vi "Ball Screw Control.vi"(6 "Target":bool, 7 "Axis":dbl, 8 "BotLimit":bool, 9 "TopLimit":bool, 10 "Closed Loop On/Off":bool, 11 "Ball Screw DevRef In":T1={"DeviceStatus"={"status"=FALSE, "code"=0, "source"=""}, "Type"=enum."PWM", "PWM"={"Digital Module"=enum."Digital Module 1", "PWM Channel"=enum."Invalid", "DeadBand"={"Name"="", "maxPositivePwm"=0, "minPositivePwm"=0, "centerPwm"=0, "maxNegativePwm"=0, "minNegativePwm"=0, "angularRange"=0}}, "CAN"={"Device Number"=0, "Control Mode"=enum."Percent VBus", "Semaphore"=refnum, "Max Vout"=12.0}, "Invert"=FALSE, "TransformRef"=refnum, "InvTransformRef"=refnum}) -> (2 "Motor Output":dbl, 3 "Ball Screw DevRef Out":T1={"DeviceStatus"={"status"=FALSE, "code"=0, "source"=""}, "Type"=enum."PWM", "PWM"={"Digital Module"=enum."Digital Module 1", "PWM Channel"=enum."Invalid", "DeadBand"={"Name"="", "maxPositivePwm"=0, "minPositivePwm"=0, "centerPwm"=0, "maxNegativePwm"=0, "minNegativePwm"=0, "angularRange"=0}}, "CAN"={"Device Number"=0, "Control Mode"=enum."Percent VBus", "Semaphore"=refnum, "Max Vout"=12.0}, "Invert"=FALSE, "TransformRef"=refnum, "InvTransformRef"=refnum})   [LabVIEW 2012]
uses:
  <vilib>/Rock Robotics/WPI/MotorControl/WPI_MotorControlDeviceRef.ctl
  <vilib>/Rock Robotics/SystemInterfaces/Typedef/FPGA_TypedefDigitalModule.ctl
  <vilib>/Rock Robotics/SystemInterfaces/DIO/FPGA_DIOPWMChannel.ctl
  <vilib>/Rock Robotics/WPI/PWM/WPI_PWMDeadband.ctl
  <vilib>/Rock Robotics/WPI/CAN/Jaguar/SubVIs/WPI_CANJaguar_ControlMode.ctl
  <vilib>/Rock Robotics/WPI/PWM/WPI_PWMTransform_ConPane.ctl
  <vilib>/Rock Robotics/WPI/CAN/Jaguar/SubVIs/WPI_CANJaguar_PositionReference.ctl
  Robot Global Data.vi
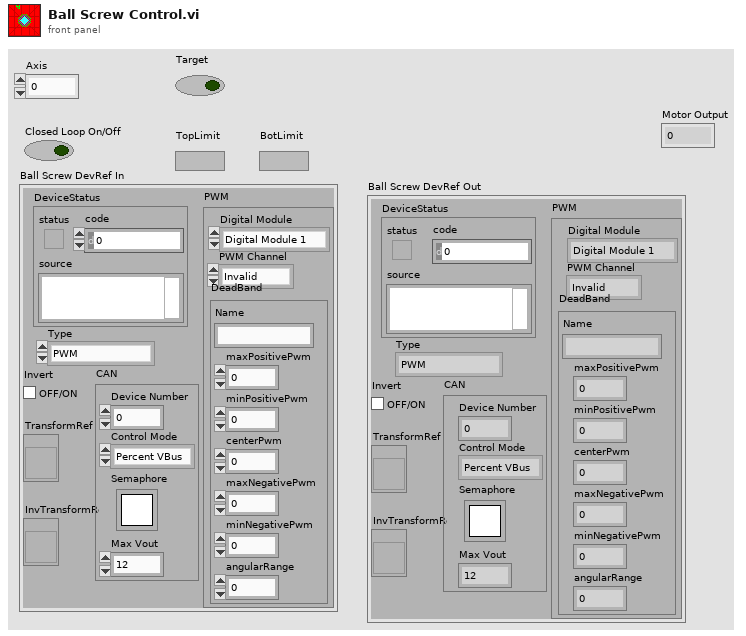
[diagram p1: front panel]
types:
  T1 = typedef "WPI_MotorControlDeviceRef.ctl" = cluster{"DeviceStatus":errorcluster, "Type":enum16{"PWM", "CAN"}, "PWM":cluster{"Digital Module":T2, "PWM Channel":T3, "DeadBand":T4}, "CAN":cluster{"Device Number":u8, "Control Mode":T5, "Semaphore":T6, "Max Vout":dbl}, "Invert":bool, "TransformRef":T7, "InvTransformRef":T7}
  T2 = typedef "FPGA_TypedefDigitalModule.ctl" = enum16{"Digital Module 1", "Digital Module 2"}
  T3 = typedef "FPGA_DIOPWMChannel.ctl" = enum8{"PWM 1", "PWM 2", "PWM 3", "PWM 4", "PWM 5", "PWM 6", "PWM 7", "PWM 8", "PWM 9", "PWM 10", "Invalid"}
  T4 = typedef "WPI_PWMDeadband.ctl" = cluster{"Name":string, "maxPositivePwm":i32, "minPositivePwm":i32, "centerPwm":i32, "maxNegativePwm":i32, "minNegativePwm":i32, "angularRange":u16}
  T5 = typedef "WPI_CANJaguar_ControlMode.ctl" = enum8{"Percent VBus", "Current", "Speed", "Position", "Voltage"}
  T6 = typedef "Semaphore RefNum" = refnum<k1>
  T7 = typedef "WPI_PWMTransform_ConPane.ctl" = refnum<vi>
  T8 = typedef "WPI_CANJaguar_PositionReference.ctl" = u8
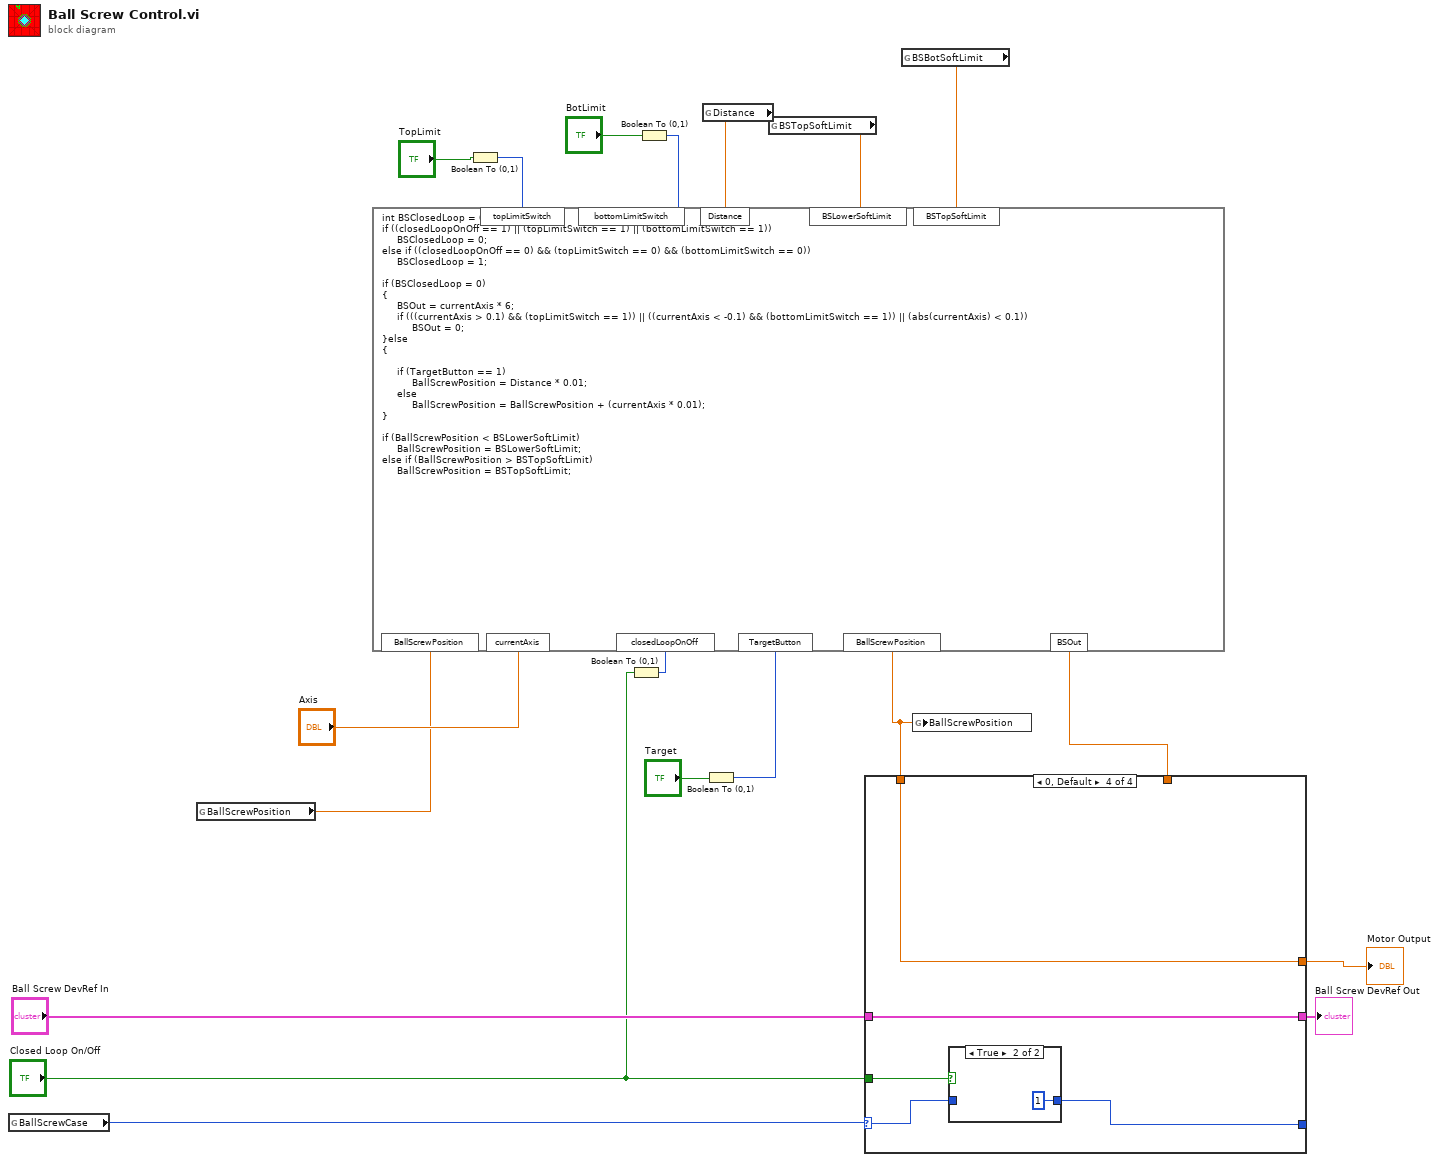
[diagram p0: block diagram]
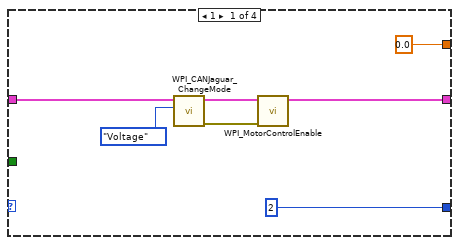
[diagram p2: hidden frame]
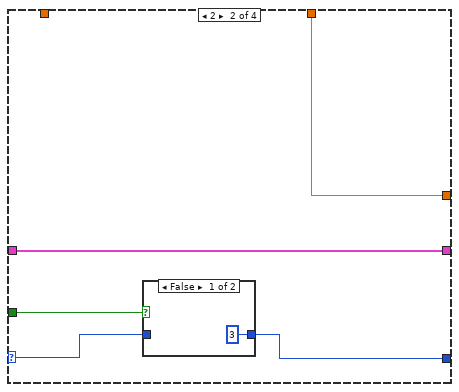
[diagram p3: hidden frame]
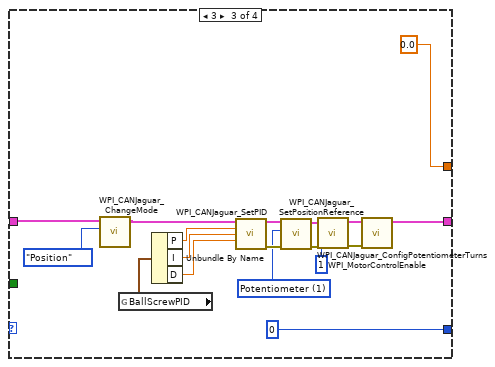
[diagram p5: hidden frame]
diagram:
  n1 = global read "Robot Global Data.vi" "BallScrewCase"() -> (w19:i8)
  n2 = global read "Robot Global Data.vi" "BallScrewPosition"() -> (w7:dbl)
  n3 = Boolean To (0,1)(Boolean="TopLimit") -> (0, 1=w14:i16)
  n4 = Boolean To (0,1)(Boolean="Closed Loop On/Off") -> (0, 1=w16:i16)
  n5 = Boolean To (0,1)(Boolean="BotLimit") -> (0, 1=w12:i16)
  n6 = global read "Robot Global Data.vi" "Distance"() -> (w6:dbl)
  n7 = Boolean To (0,1)(Boolean="Target") -> (0, 1=w9:i16)
  n8 = global read "Robot Global Data.vi" "BSTopSoftLimit"() -> (w5:dbl)
  n9 = global read "Robot Global Data.vi" "BSBotSoftLimit"() -> (w4:dbl)
  n10 = formula code="int BSClosedLoop = 0;\nif ((closedLoopOnOff == 1) || (topLimitSwitch == 1) || (bottomLimitSwitch == 1))\n     BSClosedLoop = 0;\nelse if ((closedLoopOnOff == 0) && (topLimitSwitch == 0) && (bottomLimitSwitch == 0))\n     BSClosedLoop = 1;\n\nif (BSClosedLoop = 0)\n{\n     BSOut = currentAxis * 6;\n     if (((currentAxis > 0.1) && (topLimitSwitch == 1)) || ((currentAxis < -0.1) && (bottomLimitSwitch == 1)) || (abs(currentAxis) < 0.1))\n          BSOut = 0;\n}else\n{\n    \n     if (TargetButton == 1)\n          BallScrewPosition = Distance * 0.01;\n     else \n          BallScrewPosition = BallScrewPosition + (currentAxis * 0.01);\n}\n\nif (BallScrewPosition < BSLowerSoftLimit)\n     BallScrewPosition = BSLowerSoftLimit;\nelse if (BallScrewPosition > BSTopSoftLimit)\n     BallScrewPosition = BSTopSoftLimit;"("closedLoopOnOff"=w16, "topLimitSwitch"=w14, "bottomLimitSwitch"=w12, "BallScrewPosition"=w7, "currentAxis"="Axis", "TargetButton"=w9, "Distance"=w6, "BSLowerSoftLimit"=w5, "BSTopSoftLimit"=w4) -> ("BSOut"=w10:dbl, "BallScrewPosition"=w3:dbl)
  n11 = case shown="0, Default" w19 {
    selector: w19 -> [_ w29 _ w53]
    tunnel: [i8 2 ("ShooterCase") w28 i8 0 ("ShooterCase") w54] -> _
    tunnel: "Ball Screw DevRef In" -> [w25 w31 w50 w56]
    tunnel: [w21 w31 w37 w56] -> w1
    tunnel: "Closed Loop On/Off" -> [_ w30 _ w55]
    tunnel: [0.0 ("FSpeed") w27 0.0 ("FSpeed") w52] -> w2
    tunnel: w10 -> [_ w27 _ _]
    tunnel: w3 -> [_ _ _ w52]
    frame 1 {
      n12 = call <vilib>:"WPI_CANJaguar_ChangeMode.vi"("Control Mode"=WPI_CANJaguar_ControlMode."Voltage", "CAN Jaguar Ref"=w25) -> ("error out"=w22:errorcluster, "CAN Jaguar Ref Out"=w23:T1)  [unwired: 8 in]
      n13 = call <vilib>:"WPI_MotorControlEnable.vi"("error in (no error)"=w22, "CAN Jaguar Ref"=w23) -> ("CAN Jaguar Ref Out"=w21:T1)  [unwired: 8 in, 1 out]
    }
    frame 2 {
      n14 = case shown="False" w30 {
        tunnel: [i8 3 ("ShooterCase") w33] -> w28
        tunnel: w29 -> [_ w33]
        frame False {
        }
        frame True {
        }
      }
    }
    frame 3 {
      w35 = T8 1 items=["Quad Encoder"=0, "Potentiometer"=1, "None"=255] ("Position Reference")
      n15 = call <vilib>:"WPI_CANJaguar_ChangeMode.vi"("Control Mode"=WPI_CANJaguar_ControlMode."Position", "CAN Jaguar Ref"=w50) -> ("CAN Jaguar Ref Out"=w45:T1)  [unwired: 8 in, 1 out]
      n16 = global read "Robot Global Data.vi" "BallScrewPID"() -> (w49:cluster{"P":dbl, "I":dbl, "D":dbl})
      n17 = Unbundle By Name(w49) -> ("P"=w48:dbl, "I"=w47:dbl, "D"=w46:dbl)
      n18 = call <vilib>:"WPI_CANJaguar_SetPID.vi"("CAN Jaguar Ref"=w45, "P"=w48, "I"=w47, "D"=w46) -> ("CAN Jaguar Ref Out"=w43:T1, "error out"=w42:errorcluster)  [unwired: 10 in]
      n19 = call <vilib>:"WPI_CANJaguar_SetPositionReference.vi"("error in (no error)"=w42, "Position Reference"=w35, "CAN Jaguar Ref"=w43) -> ("error out"=w40:errorcluster, "CAN Jaguar Ref Out"=w41:T1)  [unwired: 7 in]
      n20 = call <vilib>:"WPI_CANJaguar_ConfigPotentiometerTurns.vi"("error in (no error)"=w40, "Potentiometer Turns"=u16 1, "CAN Jaguar Ref"=w41) -> ("error out"=w39:errorcluster, "CAN Jaguar Ref Out"=w38:T1)  [unwired: 7 in]
      n21 = call <vilib>:"WPI_MotorControlEnable.vi"("error in (no error)"=w39, "CAN Jaguar Ref"=w38) -> ("CAN Jaguar Ref Out"=w37:T1)  [unwired: 8 in, 1 out]
    }
    frame 0, Default {
      n22 = case shown="True" w55 {
        tunnel: [w57 i8 1 ("ShooterCase")] -> w54
        tunnel: w53 -> [w57 _]
        frame False {
        }
        frame True {
        }
      }
    }
  }
  "Motor Output" <- w2
  "Ball Screw DevRef Out" <- w1
  n23 = global write "Robot Global Data.vi" "BallScrewPosition"(w3) -> ()
